vi "Waveform formatting.vi"(1 "Cluster":T1={"Closed Loop Enabled"=FALSE, "Proportional valve 1"=0.0, "Proportional valve 2"=0.0, "Controller"={"Control Algorithm"=enum."LQG-LTR", "K"={"A"=[[1.62451, -0.722865, 0.589162, 0.0258055, -0.291247, -0.19871], [0.616764, 0.243215, 0.627021, 0.310989, -0.690401, -0.192347], [-1.01378, 1.19782, 0.595116, 0.307107, -0.873915, -0.221858], [0.460934, 0.301624, 0.892121, 0.145562, -1.07734, -0.276248], [-0.148448, 0.409634, 0.289356, 0.289437, -0.348463, -0.146062], [-0.46568, 0.0291416, 0.0291565, 0.00664228, 0.274253, 0.0367555]], "B"=[[-0.400941, 1.75732], [-0.839249, -0.493575], [-1.18504, -0.379909], [-0.825179, 0.0646258], [0.655259, -0.107787], [0.351957, -0.140832]], "C"=[[0.185781, 0.5585, 1.12711, -0.0910001, -2.59125, -0.578566], [-1.86119, 1.94847, -1.12933, 0.309409, -0.22228, -0.226668]], "D"=[[4.45609, -0.0220273], [-0.0283496, 4.51922]]}, "PI/W1"={"A"=[[-4.94989, 0.0218181, -352.966, 23.8192, -3.10685, -0.000952287], [-0.0218181, -4.904857, 23.4819, -343.472, 0.000977323, -3.58066], [0.0389045, 0.0, -31.6573, 0.0287797, 0.0245405, 0.0], [0.0, 0.0381972, 0.0287797, -31.6573, 0.0, 0.0280468], [0.0, 0.0325383, 0.0240248, -0.0293675, -0.0245405, 0.0], [0.031831, 0.0, -0.0282058, 0.0, 0.0, 0.0]], "B"=[[28.0692, -23.9099], [-23.3912, 28.5852], [31.6468, -0.0287797], [-0.0287797, 31.6468], [-0.0282058, -0.0293675], [0.0282058, -0.0240214]], "C"=[[4.94989, 0.0218181, 314.896, 0.0907351, 3.10685, 0.000952287], [10.0218181, 4.90457, -0.0906726, 314.884, -0.000977323, 3.58066]], "D"=[[0.0, 0.0], [0.0, 0.0]]}, "W2"={"A"=[[-4.94989, 0.0218181, -352.966, 23.8192, -3.10685, -0.000952287], [-0.0218181, -4.904857, 23.4819, -343.472, 0.000977323, -3.58066], [0.0389045, 0.0, -31.6573, 0.0287797, 0.0245405, 0.0], [0.0, 0.0381972, 0.0287797, -31.6573, 0.0, 0.0280468], [0.0, 0.0325383, 0.0240248, -0.0293675, -0.0245405, 0.0], [0.031831, 0.0, -0.0282058, 0.0, 0.0, 0.0]], "B"=[[28.0692, -23.9099], [-23.3912, 28.5852], [31.6468, -0.0287797], [-0.0287797, 31.6468], [-0.0282058, -0.0293675], [0.0282058, -0.0240214]], "C"=[[4.94989, 0.0218181, 314.896, 0.0907351, 3.10685, 0.000952287], [10.0218181, 4.90457, -0.0906726, 314.884, -0.000977323, 3.58066]], "D"=[[0.0, 0.0], [0.0, 0.0]]}}, "Setpoint"={"Setpoints"={"Setpoint Tank 1"=0.0, "Setpoint Tank 2"=0.0, "Sin on-off"=enum."On", "Amplitude Tank 1"=0.0, "Amplitude Tank 2"=0.0, "Frequency Tank 1"=0.0, "Frequency Tank 2"=0.0, "Phase Tank 1"=0.0, "Phase Tank 2"=0.0}, "Disturbance"={"Distubance pump 1"=FALSE, "Amplitude Pump 1"=0.0, "Distubance pump 2"=FALSE, "Amplitude Pump 2"=0.0}}, "Plant Control Variables"={"Tank 1 Level"=0.0, "Tank 2 Level"=0.0, "Tank 3 Level"=0.0, "Tank 4 Level"=0.0, "Pump 1"=0.0, "Pump 2"=0.0, "Setpoint 1 signal"=0.0, "Setpoint 2 signal"=0.0}}) -> (0 "Tank Levels":waveform(dbl)[](array[waveform]))   [LabVIEW 2020]
uses:
  Real-Time/controls/Controller Data.ctl
  Real-Time/Control Algorithm/Control Algorithm Data.ctl
  Real-Time/Control Algorithm/Control Algorithm Selection.ctl
  controls/Setpoints.ctl
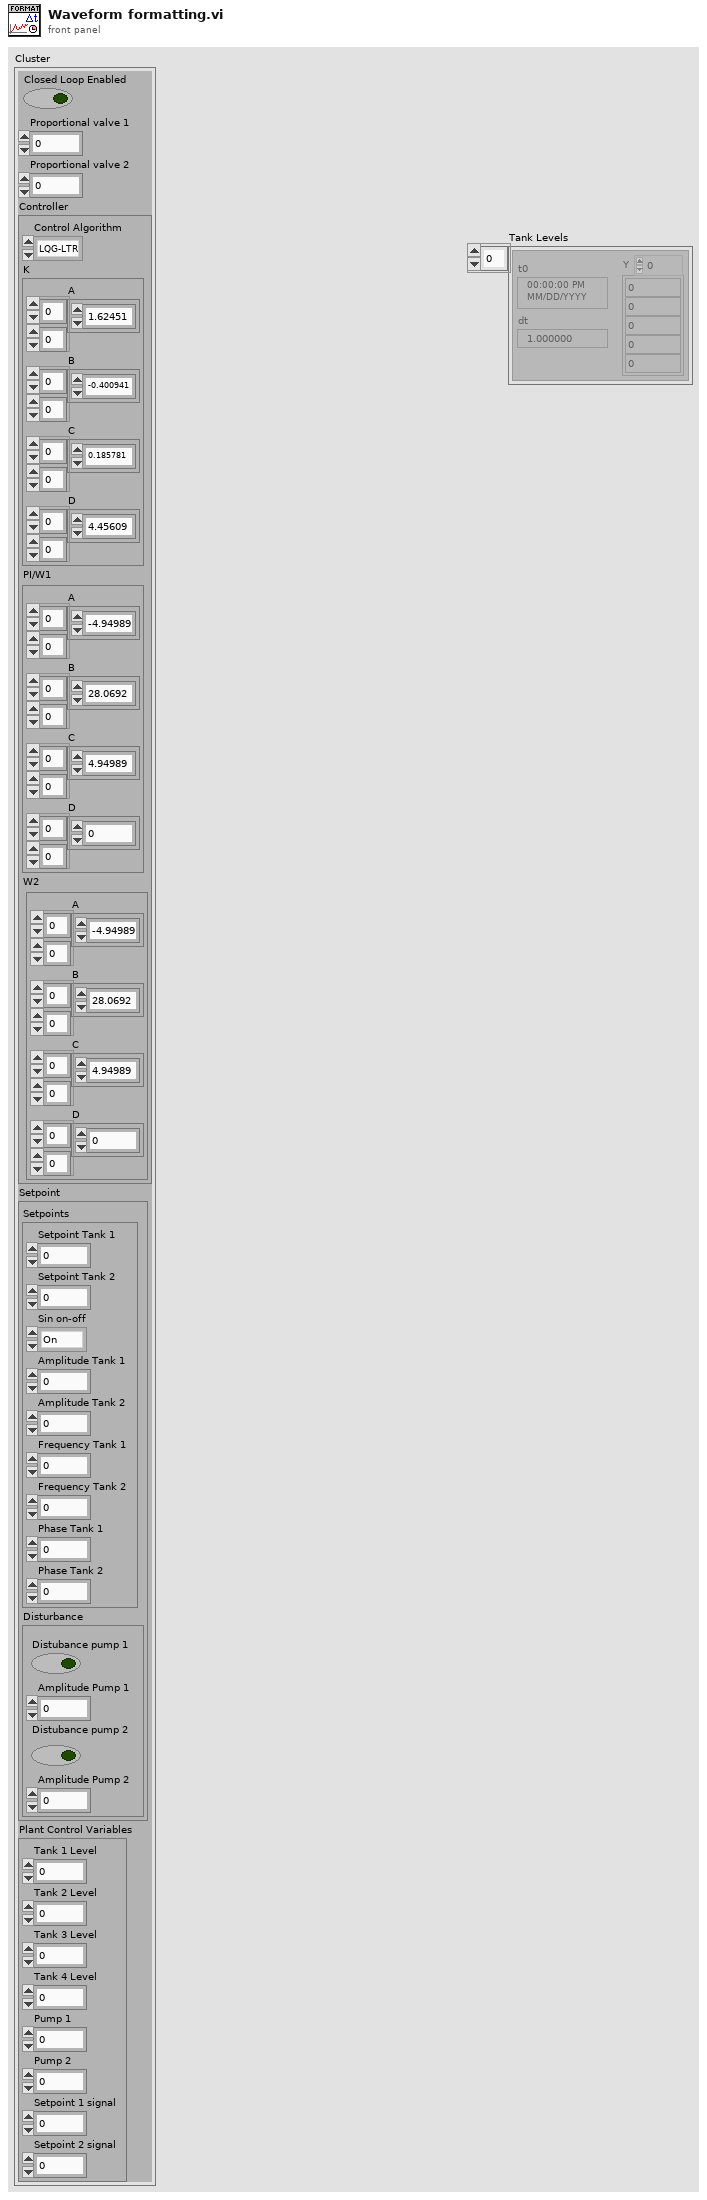
[diagram p1: front panel]
types:
  T1 = typedef "Controller Data.ctl" = cluster{"Closed Loop Enabled":bool, "Proportional valve 1":dbl, "Proportional valve 2":dbl, "Controller":T2, "Setpoint":T4, "Plant Control Variables":cluster{"Tank 1 Level":dbl, "Tank 2 Level":dbl, "Tank 3 Level":dbl, "Tank 4 Level":dbl, "Pump 1":dbl, "Pump 2":dbl, "Setpoint 1 signal":dbl, "Setpoint 2 signal":dbl}}
  T2 = typedef "Control Algorithm Data.ctl" = cluster{"Control Algorithm":T3, "K":cluster{"A":dbl[][], "B":dbl[][], "C":dbl[][], "D":dbl[][]}, "PI/W1":cluster{"A":dbl[][], "B":dbl[][], "C":dbl[][], "D":dbl[][]}, "W2":cluster{"A":dbl[][], "B":dbl[][], "C":dbl[][], "D":dbl[][]}}
  T3 = typedef "Control Algorithm Selection.ctl" = enum16{"LQG-LTR", "Hinf", "New Controller"}
  T4 = typedef "Setpoints.ctl" = cluster{"Setpoints":cluster{"Setpoint Tank 1":dbl, "Setpoint Tank 2":dbl, "Sin on-off":enum32{"On", "Off"}, "Amplitude Tank 1":dbl, "Amplitude Tank 2":dbl, "Frequency Tank 1":dbl, "Frequency Tank 2":dbl, "Phase Tank 1":dbl, "Phase Tank 2":dbl}, "Disturbance":cluster{"Distubance pump 1":bool, "Amplitude Pump 1":dbl, "Distubance pump 2":bool, "Amplitude Pump 2":dbl}}
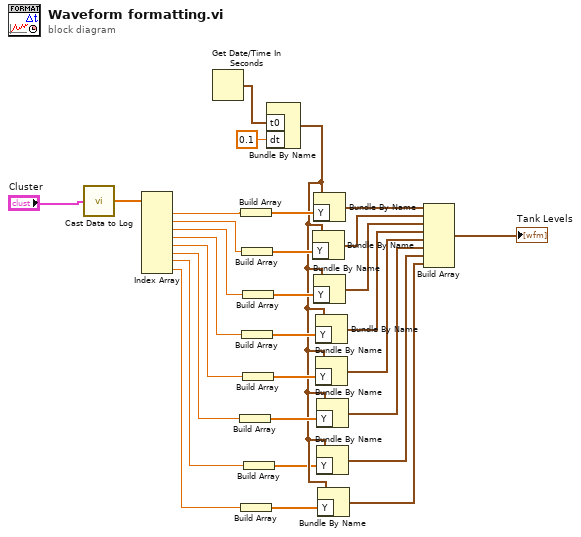
[diagram p0: block diagram]
diagram:
  n1 = call "Cast Data to Log.vi"("Data in"="Cluster") -> ("Data out"=w2:dbl[])  [unwired: 4 in]
  n2 = Index Array(array=w2) -> (element #1=w26:dbl, element #2=w24:dbl, element #3=w23:dbl, element #4=w21:dbl, element #5=w19:dbl, element #6=w17:dbl, element #7=w6:dbl, element #8=w5:dbl)  [unwired: 8 in]
  n3 = Get Date/Time In Seconds() -> (seconds since 1Jan1904=w29:timestamp)
  n4 = Build Array(w17) -> (w16:dbl[])
  n5 = Build Array(w26) -> (w27:dbl[])
  n6 = Build Array(w5) -> (w9:dbl[])
  n7 = Build Array(w24) -> (w25:dbl[])
  n8 = Build Array(w21) -> (w20:dbl[])
  n9 = Build Array(w23) -> (w22:dbl[])
  n10 = Build Array(w19) -> (w18:dbl[])
  n11 = Build Array(w6) -> (w7:dbl[])
  n12 = Bundle By Name("t0"=w29, "dt"=0.1) -> (w8:waveform(dbl))  [unwired: 1 in]
  n13 = Bundle By Name(cluster=w8, "Y"=w25) -> (w10:waveform(dbl))
  n14 = Bundle By Name(cluster=w8, "Y"=w27) -> (w11:waveform(dbl))
  n15 = Bundle By Name(cluster=w8, "Y"=w22) -> (w30:waveform(dbl))
  n16 = Bundle By Name(cluster=w8, "Y"=w20) -> (w28:waveform(dbl))
  n17 = Bundle By Name(cluster=w8, "Y"=w18) -> (w15:waveform(dbl))
  n18 = Bundle By Name(cluster=w8, "Y"=w16) -> (w14:waveform(dbl))
  n19 = Bundle By Name(cluster=w8, "Y"=w7) -> (w4:waveform(dbl))
  n20 = Bundle By Name(cluster=w8, "Y"=w9) -> (w3:waveform(dbl))
  n21 = Build Array(w11, w10, w30, w28, w15, w14, w4, w3) -> (→"Tank Levels":waveform(dbl)[])
